vi "Trivial reply example.vi"() -> ()   [LabVIEW 2018]
uses:
  <vilib>/addons/zeromq/socket_type.ctl
  <vilib>/addons/zeromq/zmq_context.lvclass
  <vilib>/addons/zeromq/zmq_socket.lvclass
  <vilib>/addons/zeromq/zeromq.lvlib
panel:
  in  "endpoint":string="tcp://127.0.0.1:5555"
  out "status":string
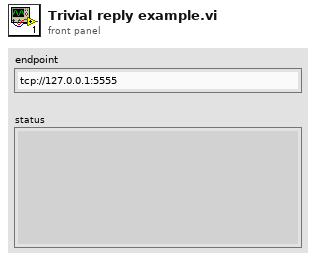
[diagram p1: front panel]
types:
  T1 = typedef "zeromq.lvlib/socket_type.ctl" = enum8{"ZMQ_PAIR", "ZMQ_PUB", "ZMQ_SUB", "ZMQ_REQ", "ZMQ_REP", "ZMQ_DEALER", "ZMQ_ROUTER", "ZMQ_PULL", "ZMQ_PUSH", "ZMQ_XPUB", "ZMQ_XSUB", "ZMQ_STREAM", "ZMQ_SERVER", "ZMQ_CLIENT", "ZMQ_RADIO", "ZMQ_DISH", "ZMQ_GATHER", "ZMQ_SCATTER", "ZMQ_DGRAM"}
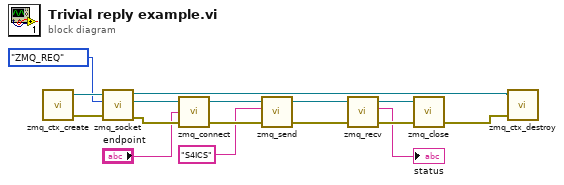
[diagram p0: block diagram]
diagram:
  n1 = call <vilib>:"zmq_ctx_create.vi"() -> ("error out"=w15:errorcluster, "context out"=w16:refnum<class "zmq_context.lvclass">)  [unwired: 4 in]
  n2 = call <vilib>:"zmq_socket.vi"("error in"=w15, "socket type"=socket_type."ZMQ_REQ", "context in"=w16) -> ("error out"=w13:errorcluster, "socket out"=w5:refnum<class "zmq_socket.lvclass">, "context out"=w14:refnum<class "zmq_context.lvclass">)  [unwired: 2 in]
  n3 = call <vilib>:"zmq_connect.vi"("error in"=w13, "endpoint"="endpoint", "socket in"=w5) -> ("error out"=w6:errorcluster, "socket out"=w12:refnum<class "zmq_socket.lvclass">)  [unwired: 1 in]
  n4 = call <vilib>:"zmq_send.vi"("error in"=w6, "data"="S4ICS", "socket in"=w12) -> ("error out"=w7:errorcluster, "socket out"=w11:refnum<class "zmq_socket.lvclass">)  [unwired: 4 in]
  n5 = call <vilib>:"zmq_recv.vi"("error in"=w7, "socket in"=w11) -> ("error out"=w8:errorcluster, "data"=→"status":string, "socket out"=w10:refnum<class "zmq_socket.lvclass">)  [unwired: 3 in, 2 out]
  n6 = call <vilib>:"zmq_close.vi"("error in"=w8, "socket"=w10) -> ("error out"=w9:errorcluster)  [unwired: 3 in]
  n7 = call <vilib>:"zmq_ctx_destroy.vi"("error in"=w9, "context in"=w14) -> ()  [unwired: 3 in, 1 out]
